vi "CHD_ODOM_BEGIN.vi"(8 "error in (no error)":errorcluster, 9 "Initial Pose":T1={"TRANSLATION"={"X"=2.0, "Y"=4.0}, "ROTATION"={"VALUE"=0.0, "COS"=0.0, "SIN"=0.0}} {"ROTATION"."SIN" format="%13.4f"; "ROTATION"."COS" format="%13.4f"; "ROTATION"."VALUE" format="%13.4f"; "TRANSLATION"."Y" format="%14.3f"; "TRANSLATION"."X" format="%14.3f"}, 10 "Initial Gyro Angle":T3 {"SIN" format="%13.4f"; "COS" format="%13.4f"; "VALUE" format="%13.4f"}) -> (0 "error out":errorcluster)   [LabVIEW 2019]
uses:
  <vilib>/Rock Robotics/WPI/ThirdParty/JAS_Junk/TrajLib/Trajectory_Library.lvlib
  <vilib>/Rock Robotics/WPI/ThirdParty/JAS_Junk/TrajLib/TypeDef/ROTATION2D.ctl
  <vilib>/Rock Robotics/WPI/ThirdParty/JAS_Junk/TrajLib/TypeDef/TRANSLATION2D.ctl
  <vilib>/Rock Robotics/WPI/ThirdParty/JAS_Junk/TrajLib/TypeDef/POSE2D.ctl
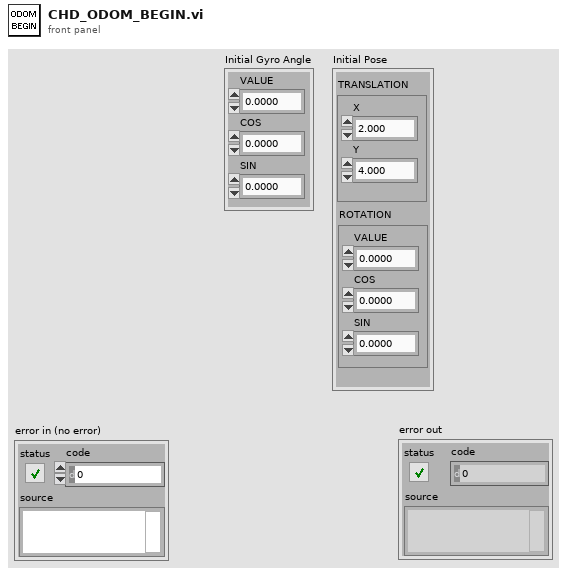
[diagram p1: front panel]
types:
  T1 = typedef "Trajectory_Library.lvlib/POSE2D.ctl" = cluster{"TRANSLATION":T2, "ROTATION":T3}
  T2 = typedef "Trajectory_Library.lvlib/TRANSLATION2D.ctl" = cluster{"X":dbl, "Y":dbl}
  T3 = typedef "Trajectory_Library.lvlib/ROTATION2D.ctl" = cluster{"VALUE":dbl, "COS":dbl, "SIN":dbl}
  T4 = typedef "Trajectory_Library.lvlib/DIFF_DRIVE_ODOM2.ctl" = cluster{"M_POSE_Meters":T1, "M_GyroOffset":T3, "M_PrevAngle":T3, "M_PrevLeftDist_M":dbl, "M_PrevRightDist_M":dbl, "M_InitLeftDist_M":dbl, "M_InitRightDist_M":dbl}
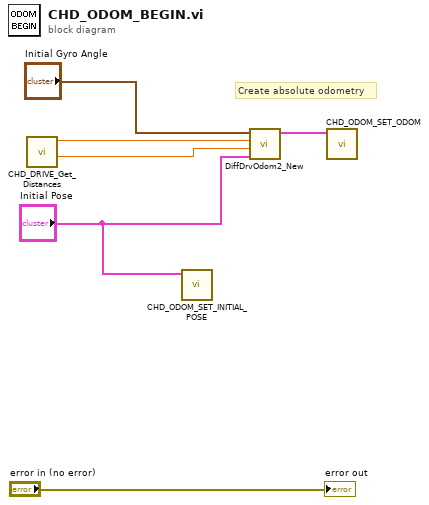
[diagram p0: block diagram]
diagram:
  # "Create absolute odometry"
  n1 = call "CHD_DRIVE_Get_Distances.vi"() -> ("RightDistance_M"=w3:dbl, "LeftDistance_M"=w4:dbl)  [unwired: 9 in, 1 out]
  n2 = call "CHD_ODOM_SET_INITIAL_POSE.vi"("Initial Odometry Pose"="Initial Pose") -> ()  [unwired: 11 in]
  n3 = call <vilib>:"DiffDrvOdom2_New.vi"("Initial Pose Meters"="Initial Pose", "Initial Right Distance M"=w3, "Initial Left Distance M"=w4, "Initial Gyro Reading"="Initial Gyro Angle") -> ("Out DIFF_DRIVE_ODOM"=w2:T4)  [unwired: 7 in]
  n4 = call "CHD_ODOM_SET_ODOM.vi"("Absolue Odometry"=w2) -> ()  [unwired: 11 in]
  "error out" <- "error in (no error)"
